vi "DecodeWordsFromPic.vi"(10 "AfterRecombinedData":u8[](array[numeric]), 11 "String":string) -> (2 "Decoded String":string, 3 "Decoded Words Size":i32)   [LabVIEW 2016]
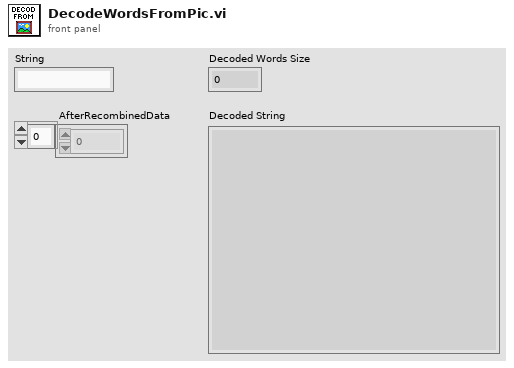
[diagram p1: front panel]
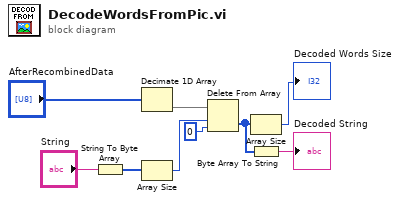
[diagram p0: block diagram]
diagram:
  n1 = String To Byte Array(string="String") -> (unsigned byte array=w5:u8[])
  n2 = Decimate 1D Array("AfterRecombinedData") -> (w8:u8[])  [unwired: 2 out]
  n3 = Array Size(array=w5) -> (size(s)=w7:i32)
  n4 = Delete From Array(array=w8, length=w7, index=0) -> (deleted portion=w3:u8[])  [unwired: 1 out]
  n5 = Array Size(array=w3) -> (size(s)=→"Decoded Words Size":i32)
  n6 = Byte Array To String(unsigned byte array=w3) -> (string=→"Decoded String":string)
